vi "RunPythonProcessData.vi"(9 "Compiler Settings":T1={"Python Path"=path "", "Main File"="mainscript.py", "Meta File"="metascript.txt", "Aux File"="auxscript.py", "Pre File"="metascript.txt"}, 11 "filepath":string) -> (2 "standard error":string, 3 "standard output":string)   [LabVIEW 2019]
uses:
  PulseCompiler/CompilerSettings.ctl
panel:
  in  "error in (no error)":errorcluster
  out "error out":errorcluster
  out "return code":i32
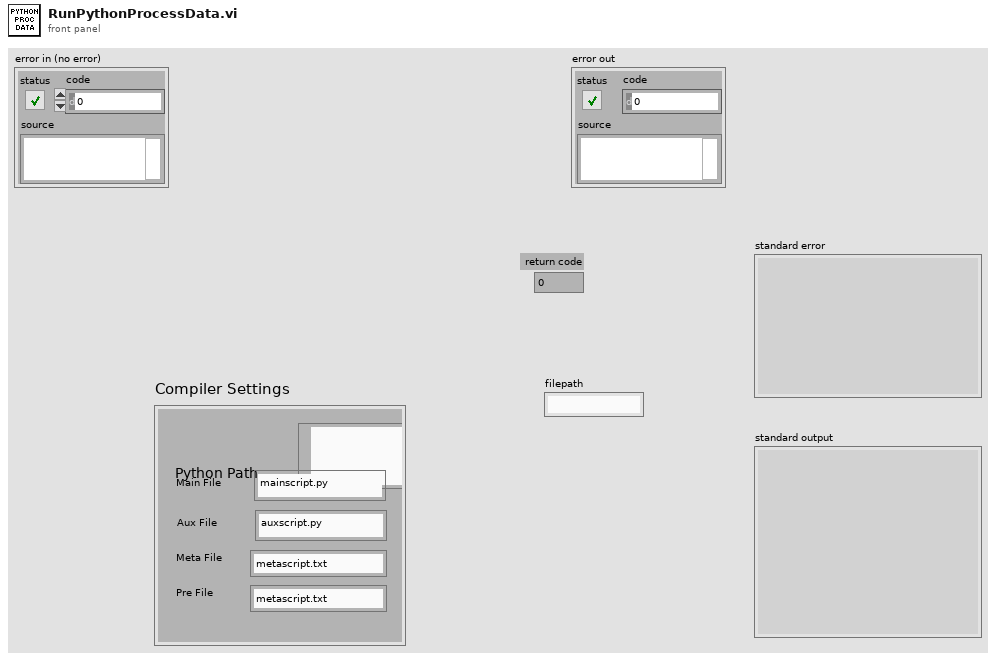
[diagram p1: front panel]
types:
  T1 = typedef "CompilerSettings.ctl" = cluster{"Python Path":path, "Main File":string, "Meta File":string, "Aux File":string, "Pre File":string}
  T2 = cluster{"filepath":string, "calib":i32, "genimage":i32}
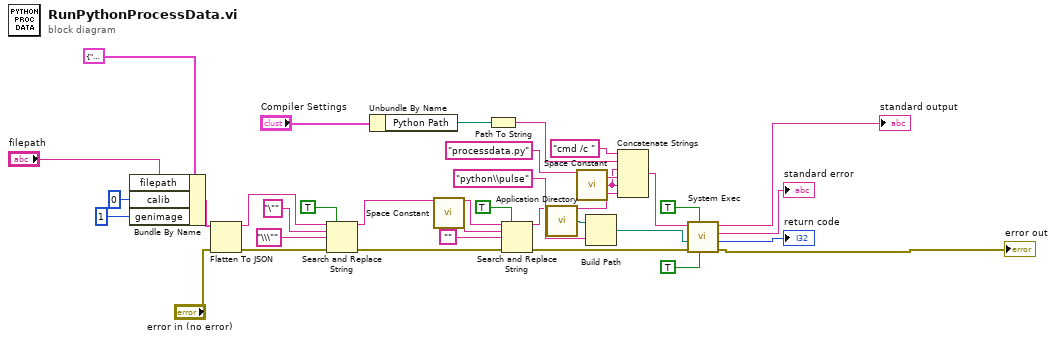
[diagram p0: block diagram]
diagram:
  n1 = Bundle By Name(cluster=T2 {"filepath"="", "calib"=0, "genimage"=1}, "filepath"="filepath", "calib"=0, "genimage"=1) -> (w8:T2)
  n2 = Flatten To JSON(anything=w8, error in (no error)="error in (no error)") -> (JSON string=w21:string, 11:w20:errorcluster)  [unwired: 1 in]
  n3 = Search and Replace String(replace all?=TRUE ("replace all? (F)"), input string=w21, search string="\"", replace string="\\\"" ("replace string (\"\")"), error in=w20) -> (result string=w17:string, error out=w16:errorcluster)  [unwired: 3 in, 2 out]
  n4 = Unbundle By Name("Compiler Settings") -> ("Python Path"=w7:path)
  n5 = call <vilib>:"Space Constant.vi"() -> ("String"=w15:string)
  n6 = Path To String(path=w7) -> (string=w6:string)
  n7 = Search and Replace String(replace all?=TRUE ("replace all? (F)"), input string=w17, search string=w15, replace string="", error in=w16) -> (result string=w13:string, error out=w12:errorcluster)  [unwired: 3 in, 2 out]
  n8 = call <vilib>:"Application Directory.vi"() -> ("Application Directory"=w25:path)
  n9 = call <vilib>:"Space Constant.vi"() -> ("String"=w22:string)
  n10 = Build Path(base path=w25, name or relative path="python\\pulse") -> (appended path=w27:path)
  n11 = Concatenate Strings("cmd /c " ("string"), w6, w22, "processdata.py" ("name or relative path"), w22, w13) -> (w24:string)
  n12 = call <vilib>:"System Exec.vi"("run minimized? (F)"=TRUE, "wait until completion? (T)"=TRUE, "error in (no error)"=w12, "working directory"=w27, "command line"=w24) -> ("error out"=→"error out":errorcluster, "return code"=→"return code":i32, "standard error"=→"standard error":string, "standard output"=→"standard output":string)  [unwired: 3 in]
